vi "raghu rbl main online.vi"() -> ()   [LabVIEW 2015]
panel:
  out "uneven inner":bool
  out "even inner outer":bool
  out "even inner":bool
  out "brake oil spil":bool
  out "reservoir leak":bool
  out "uneven inner outer":bool
  out "good":bool
  in  "STOP":bool
  out "BOS":i32
  out "RL":i32
  out "UNEVEN IO":i32
  out "UNEVEN I":i32
  out "EVEN IO":i32
  out "EVEN I":i32
  out "G1":i32
  out "EVEN INNER OUTER":bool
  out "EVEN INNER":bool
  out "BREAK OIL SPIL":bool
  out "RESERVOIR LEAK":bool
  out "UNEVEN INNER":bool
  out "UNEVEN INNER OUTER":bool
  out "GOOD":bool
  out "Range":dbl
  out "Skewness":dbl
  out "Kurtosis":dbl
  out "Standard Dev":dbl
  # "STASTICTIAL FEATURES \nRANGES"
  # "FAULT ERROR \nREADINGS"
  # "FAULTS \nBOLENA LAMPS"
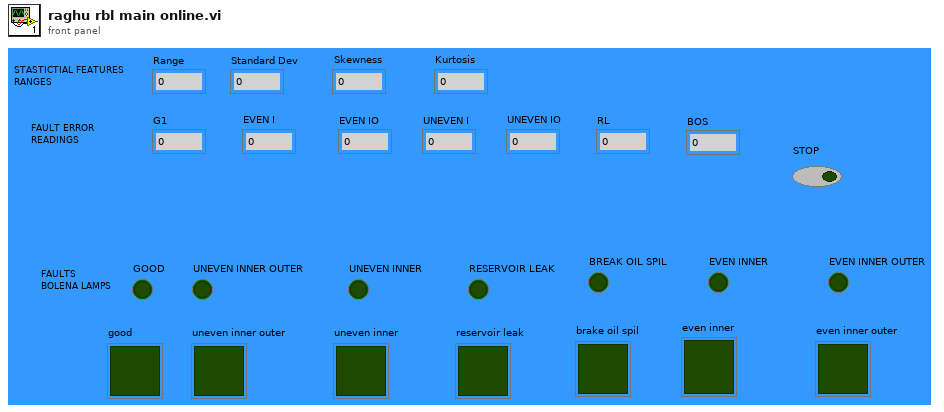
[diagram p1: front panel]
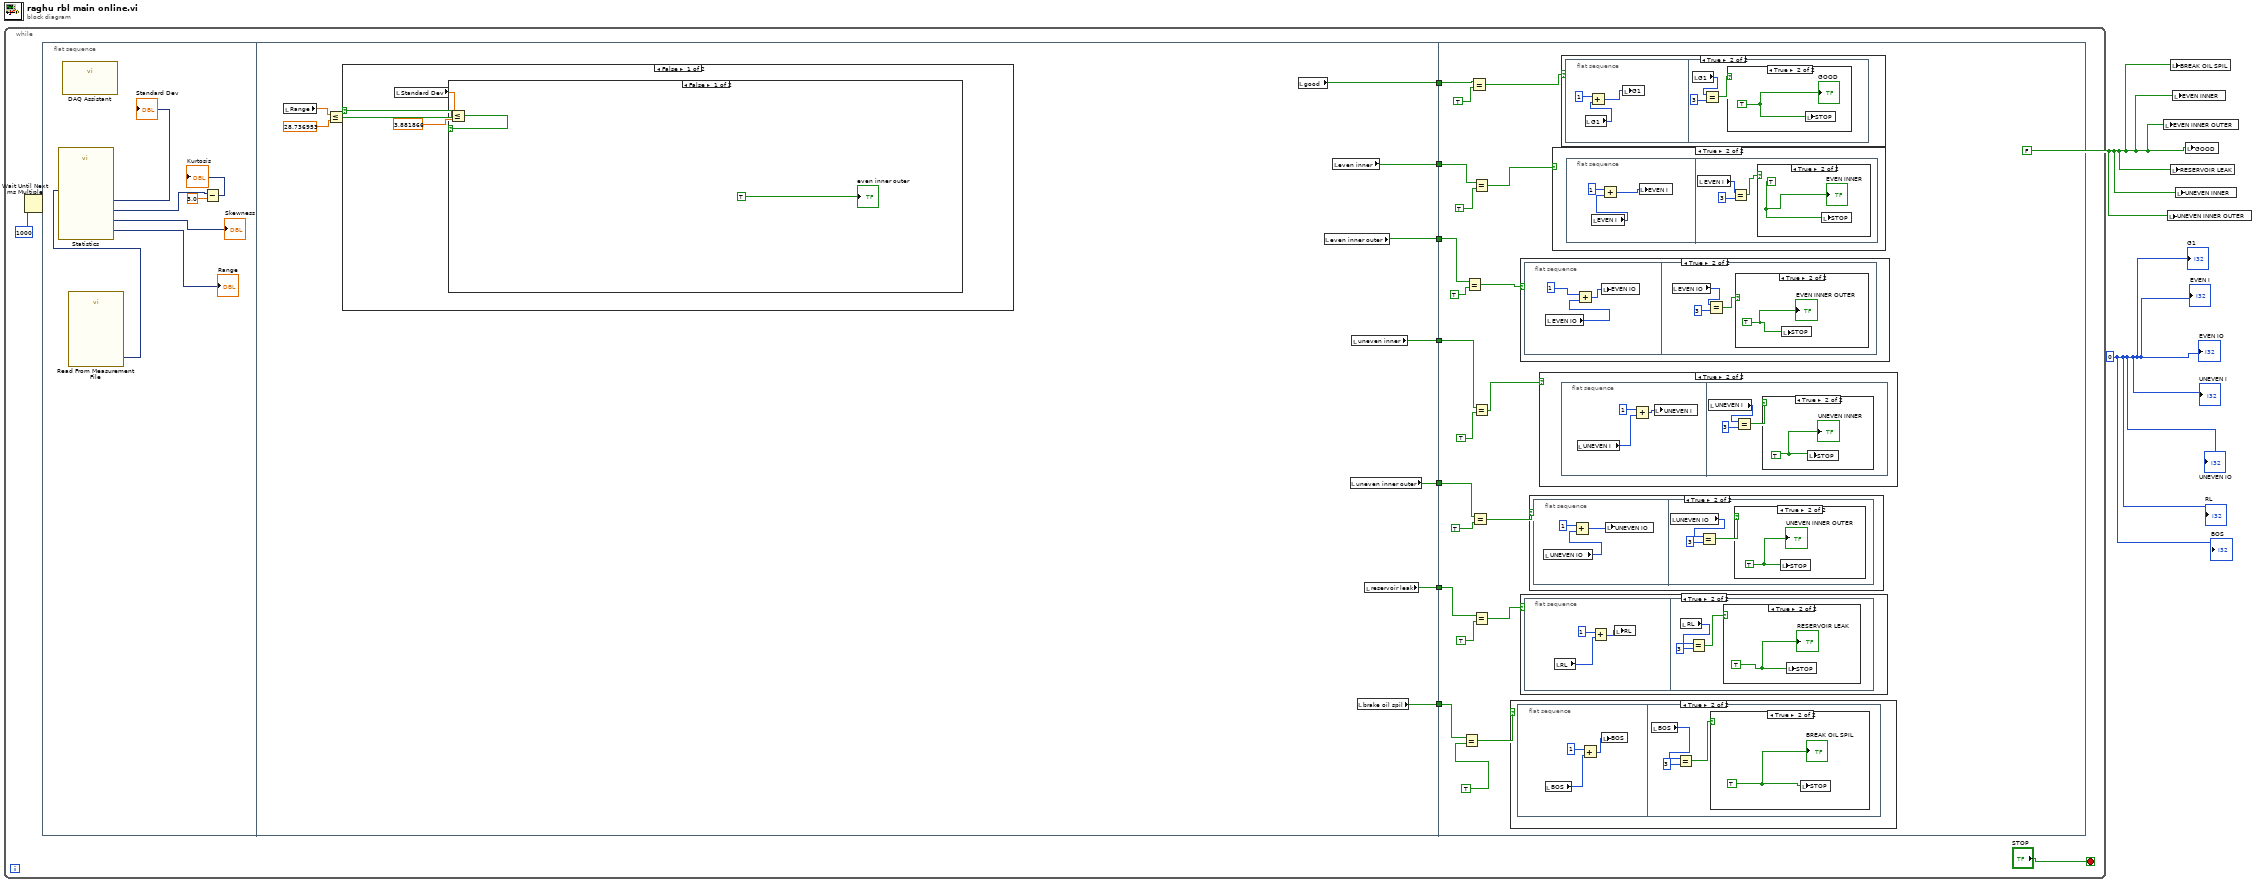
[diagram p0: block diagram]
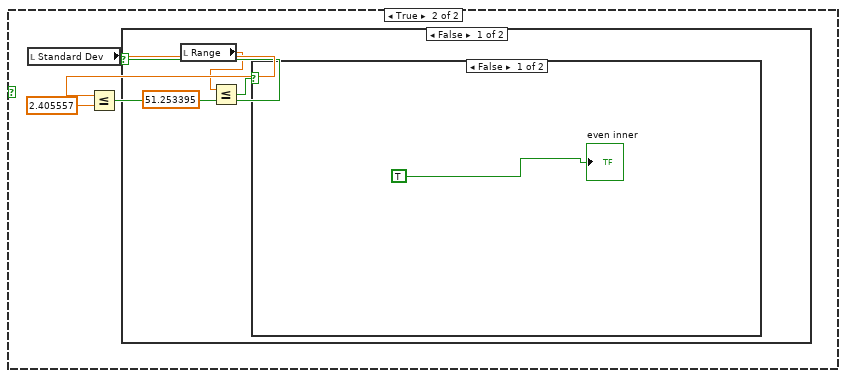
[diagram p2: hidden frame]
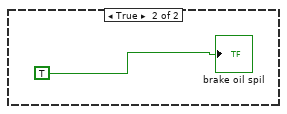
[diagram p3: hidden frame]
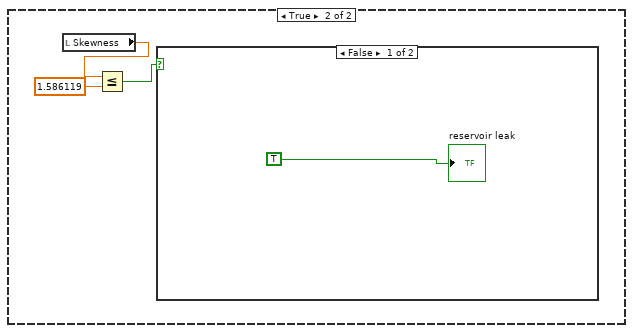
[diagram p4: hidden frame]
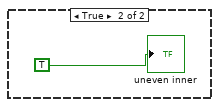
[diagram p5: hidden frame]
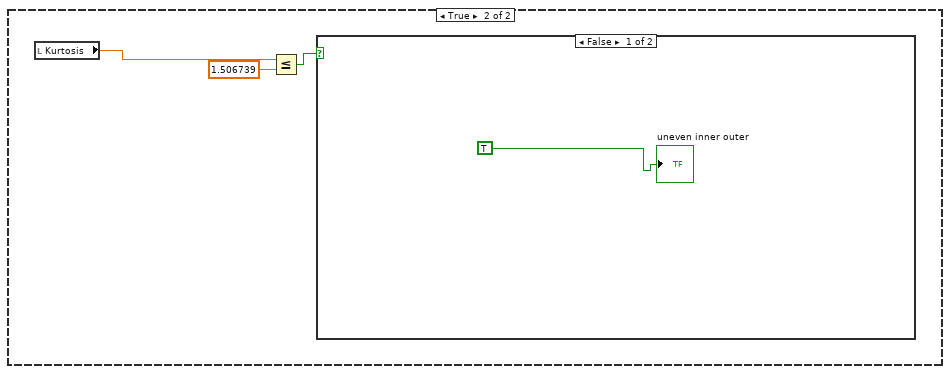
[diagram p6: hidden frame]
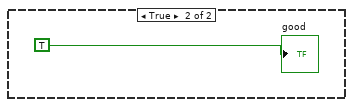
[diagram p7: hidden frame]
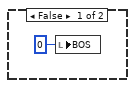
[diagram p8: hidden frame]
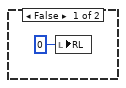
[diagram p10: hidden frame]
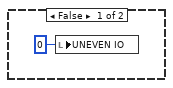
[diagram p12: hidden frame]
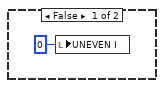
[diagram p14: hidden frame]
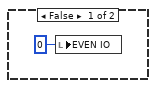
[diagram p16: hidden frame]
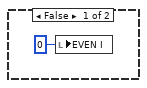
[diagram p18: hidden frame]
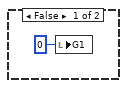
[diagram p20: hidden frame]
diagram:
  w1 = 0
  w2 = FALSE
  n1 = while {
    stop <- "STOP" stop-if-true
    n2 = Wait Until Next ms Multiple(millisecond multiple=u32 1000) -> ()  [unwired: 1 out]
    n3 = flat-sequence {
      tunnel: [w28] -> w10
      tunnel: [w27] -> w9
      tunnel: [w26] -> w8
      tunnel: [w25] -> w7
      tunnel: [w24] -> w6
      tunnel: [w23] -> w5
      tunnel: [w22] -> w3
      tunnel: w10 -> [w69]
      tunnel: w9 -> [w67]
      tunnel: w8 -> [w64]
      tunnel: w7 -> [w61]
      tunnel: w6 -> [w58]
      tunnel: w5 -> [w55]
      tunnel: w3 -> [w51]
      frame #0 {
        n4 = call "DAQ Assistant"() -> ()  [unwired: 12 in]
        n5 = call "Read From Measurement File"() -> ("Signals"=w12:dynamicdata)  [unwired: 6 in, 5 out]
        n6 = call "Statistics"("Signals"=w12) -> ("Skewness"=→"Skewness":dynamicdata, "Kurtosis"=w17:dynamicdata, "Standard Dev"=→"Standard Dev":dynamicdata, "Range"=→"Range":dynamicdata)  [unwired: 22 in, 1 out]
        n7 = Subtract(x=w17, y=3.0) -> (x-y=→"Kurtosis":dynamicdata)
      }
      frame #1 {
        n8 = local read "Range"() -> (w20:dbl)
        n9 = Less Or Equal?(x=w20, y=28.736953) -> (x <= y?=w21:bool)
        n10 = case shown="False" w21 {
          frame False {
            n11 = local read "Standard Dev"() -> (w30:dbl)
            n12 = Less Or Equal?(x=w30, y=3.881866) -> (x <= y?=w31:bool)
            n13 = case shown="False" w31 {
              frame False {
                "even inner outer" <- TRUE
              }
              frame True {
                n14 = local read "Standard Dev"() -> (w35:dbl)
                n15 = Less Or Equal?(x=w35, y=2.405557) -> (x <= y?=w34:bool)
                n16 = case shown="False" w34 {
                  frame False {
                    n17 = local read "Range"() -> (w37:dbl)
                    n18 = Less Or Equal?(x=w37, y=51.253395) -> (x <= y?=w38:bool)
                    n19 = case shown="False" w38 {
                      frame False {
                        "even inner" <- TRUE
                      }
                      frame True {
                        "brake oil spil" <- TRUE
                      }
                    }
                  }
                  frame True {
                    n20 = local read "Skewness"() -> (w42:dbl)
                    n21 = Less Or Equal?(x=w42, y=1.586119) -> (x <= y?=w43:bool)
                    n22 = case shown="False" w43 {
                      frame False {
                        "reservoir leak" <- TRUE
                      }
                      frame True {
                        "uneven inner" <- TRUE
                      }
                    }
                  }
                }
              }
            }
          }
          frame True {
            n23 = local read "Kurtosis"() -> (w47:dbl)
            n24 = Less Or Equal?(x=w47, y=1.506739) -> (x <= y?=w48:bool)
            n25 = case shown="False" w48 {
              frame False {
                "uneven inner outer" <- TRUE
              }
              frame True {
                "good" <- TRUE
              }
            }
          }
        }
        n26 = local read "good"() -> (w28:bool)
        n27 = local read "even inner outer"() -> (w26:bool)
        n28 = local read "even inner"() -> (w27:bool)
        n29 = local read "uneven inner outer"() -> (w24:bool)
        n30 = local read "uneven inner"() -> (w25:bool)
        n31 = local read "brake oil spil"() -> (w22:bool)
        n32 = local read "reservoir leak"() -> (w23:bool)
      }
      frame #2 {
        n33 = Equal?(x=w51, y=TRUE) -> (x = y?=w53:bool)
        n34 = Equal?(x=w64, y=TRUE) -> (x = y?=w65:bool)
        n35 = Equal?(x=w69, y=TRUE) -> (x = y?=w71:bool)
        n36 = Equal?(x=w58, y=TRUE) -> (x = y?=w59:bool)
        n37 = Equal?(x=w67, y=TRUE) -> (x = y?=w66:bool)
        n38 = Equal?(x=w61, y=TRUE) -> (x = y?=w62:bool)
        n39 = Equal?(x=w55, y=TRUE) -> (x = y?=w56:bool)
        n40 = case shown="True" w53 {
          frame False {
            n41 = local write "BOS"(0 ("BOS")) -> ()
          }
          frame True {
            n42 = flat-sequence {
              frame #0 {
                n43 = local read "BOS"() -> (w74:i32)
                n44 = Add(x=1, y=w74) -> (x+y=w75:i32)
                n45 = local write "BOS"(w75) -> ()
              }
              frame #1 {
                n46 = local read "BOS"() -> (w78:i32)
                n47 = Equal?(x=w78, y=3) -> (x = y?=w77:bool)
                n48 = case shown="True" w77 {
                  frame False {
                  }
                  frame True {
                    w79 = TRUE
                    n49 = local write "STOP"(w79) -> ()
                    "BREAK OIL SPIL" <- w79
                  }
                }
              }
            }
          }
        }
        n50 = case shown="True" w65 {
          frame False {
            n51 = local write "EVEN IO"(0 ("EVEN IO")) -> ()
          }
          frame True {
            n52 = flat-sequence {
              frame #0 {
                n53 = local read "EVEN IO"() -> (w106:i32)
                n54 = Add(x=1, y=w106) -> (x+y=w107:i32)
                n55 = local write "EVEN IO"(w107) -> ()
              }
              frame #1 {
                n56 = local read "EVEN IO"() -> (w109:i32)
                n57 = Equal?(x=w109, y=3) -> (x = y?=w110:bool)
                n58 = case shown="True" w110 {
                  frame False {
                  }
                  frame True {
                    w111 = TRUE
                    n59 = local write "STOP"(w111) -> ()
                    "EVEN INNER OUTER" <- w111
                  }
                }
              }
            }
          }
        }
        n60 = case shown="True" w56 {
          frame False {
            n61 = local write "RL"(0 ("RL")) -> ()
          }
          frame True {
            n62 = flat-sequence {
              frame #0 {
                n63 = local read "RL"() -> (w82:i32)
                n64 = Add(x=1, y=w82) -> (x+y=w83:i32)
                n65 = local write "RL"(w83) -> ()
              }
              frame #1 {
                n66 = local read "RL"() -> (w85:i32)
                n67 = Equal?(x=w85, y=3) -> (x = y?=w86:bool)
                n68 = case shown="True" w86 {
                  frame False {
                  }
                  frame True {
                    w87 = TRUE
                    n69 = local write "STOP"(w87) -> ()
                    "RESERVOIR LEAK" <- w87
                  }
                }
              }
            }
          }
        }
        n70 = case shown="True" w59 {
          frame False {
            n71 = local write "UNEVEN IO"(0 ("UNEVEN IO")) -> ()
          }
          frame True {
            n72 = flat-sequence {
              frame #0 {
                n73 = local read "UNEVEN IO"() -> (w91:i32)
                n74 = Add(x=1, y=w91) -> (x+y=w90:i32)
                n75 = local write "UNEVEN IO"(w90) -> ()
              }
              frame #1 {
                n76 = local read "UNEVEN IO"() -> (w93:i32)
                n77 = Equal?(x=w93, y=3) -> (x = y?=w94:bool)
                n78 = case shown="True" w94 {
                  frame False {
                  }
                  frame True {
                    w95 = TRUE
                    n79 = local write "STOP"(w95) -> ()
                    "UNEVEN INNER OUTER" <- w95
                  }
                }
              }
            }
          }
        }
        n80 = case shown="True" w62 {
          frame False {
            n81 = local write "UNEVEN I"(0 ("UNEVEN I")) -> ()
          }
          frame True {
            n82 = flat-sequence {
              frame #0 {
                n83 = local read "UNEVEN I"() -> (w99:i32)
                n84 = Add(x=1, y=w99) -> (x+y=w97:i32)
                n85 = local write "UNEVEN I"(w97) -> ()
              }
              frame #1 {
                n86 = local read "UNEVEN I"() -> (w101:i32)
                n87 = Equal?(x=w101, y=3) -> (x = y?=w102:bool)
                n88 = case shown="True" w102 {
                  frame False {
                  }
                  frame True {
                    w103 = TRUE
                    n89 = local write "STOP"(w103) -> ()
                    "UNEVEN INNER" <- w103
                  }
                }
              }
            }
          }
        }
        n90 = case shown="True" w66 {
          frame False {
            n91 = local write "EVEN I"(0 ("EVEN I")) -> ()
          }
          frame True {
            n92 = flat-sequence {
              frame #0 {
                n93 = local read "EVEN I"() -> (w114:i32)
                n94 = Add(x=1, y=w114) -> (x+y=w115:i32)
                n95 = local write "EVEN I"(w115) -> ()
              }
              frame #1 {
                n96 = local read "EVEN I"() -> (w117:i32)
                n97 = Equal?(x=w117, y=3) -> (x = y?=w118:bool)
                n98 = case shown="True" w118 {
                  frame False {
                  }
                  frame True {
                    w119 = TRUE
                    n99 = local write "STOP"(w119) -> ()
                    "EVEN INNER" <- w119
                  }
                }
              }
            }
          }
        }
        n100 = case shown="True" w71 {
          frame False {
            n101 = local write "G1"(0 ("G1")) -> ()
          }
          frame True {
            n102 = flat-sequence {
              frame #0 {
                n103 = local read "G1"() -> (w123:i32)
                n104 = Add(x=1, y=w123) -> (x+y=w121:i32)
                n105 = local write "G1"(w121) -> ()
              }
              frame #1 {
                n106 = local read "G1"() -> (w125:i32)
                n107 = Equal?(x=w125, y=3) -> (x = y?=w126:bool)
                n108 = case shown="True" w126 {
                  frame False {
                  }
                  frame True {
                    w127 = TRUE
                    n109 = local write "STOP"(w127) -> ()
                    "GOOD" <- w127
                  }
                }
              }
            }
          }
        }
      }
    }
  }
  n110 = local write "EVEN INNER OUTER"(w2) -> ()
  n111 = local write "UNEVEN INNER OUTER"(w2) -> ()
  n112 = local write "BREAK OIL SPIL"(w2) -> ()
  n113 = local write "RESERVOIR LEAK"(w2) -> ()
  n114 = local write "EVEN INNER"(w2) -> ()
  n115 = local write "UNEVEN INNER"(w2) -> ()
  n116 = local write "GOOD"(w2) -> ()
  "G1" <- w1
  "EVEN I" <- w1
  "EVEN IO" <- w1
  "UNEVEN I" <- w1
  "UNEVEN IO" <- w1
  "RL" <- w1
  "BOS" <- w1
